vi "test2.vi"() -> ()   [LabVIEW 2013]
uses:
  <vilib>/Utility/file.llb/Write To Spreadsheet File (string).vi
panel:
  out "appended path":path
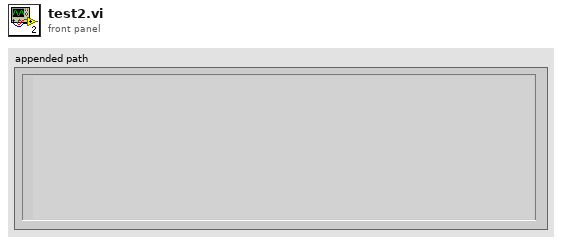
[diagram p1: front panel]
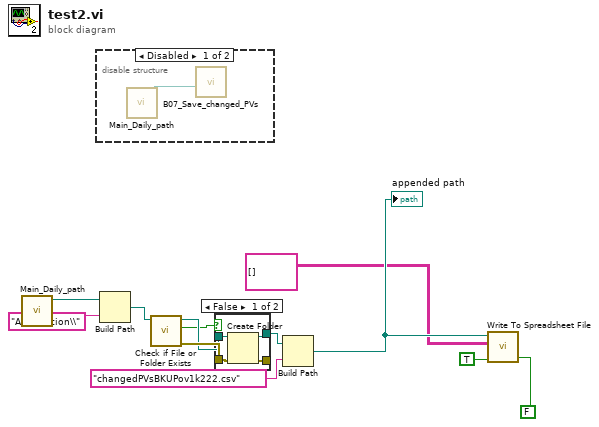
[diagram p0: block diagram]
diagram:
  n1 = call "Main_Daily_path.vi"() -> ("Directory path"=w6:path)  [unwired: 10 in, 1 out]
  n2 = disable-structure shown="Disabled" {
    frame Disabled {
      n3 = call "Main_Daily_path.vi"() -> ("Directory path"=w13:path)  [unwired: 10 in, 1 out]
      n4 = call "B07_Save_changed_PVs.vi"("Directory Path"=w13) -> ()  [unwired: 9 in, 2 out]
    }
    frame Enabled {
    }
  }
  n5 = Build Path(base path=w6, name or relative path="Association\\" ("string")) -> (appended path=w10:path)
  n6 = call <vilib>:"Check if File or Folder Exists.vi"("path"=w10) -> ("error out"=w9:errorcluster, "file or folder exists?"=w7:bool, "dup path"=w8:path)  [unwired: 8 in]
  n7 = case shown="False" w7 {
    tunnel: w8 -> [w17 w18]
    tunnel: [w16 w19] -> _
    tunnel: w9 -> [w15 w19]
    tunnel: [w14 w18] -> w11
    frame False {
      n8 = Create Folder(path (use dialog)=w17, error in=w15) -> (created path=w14:path, error out=w16:errorcluster)  [unwired: 1 in, 1 out]
    }
    frame True {
    }
  }
  n9 = Build Path(base path=w11, name or relative path="changedPVsBKUPov1k222.csv" ("string")) -> (appended path=w2:path)
  "appended path" <- w2
  n10 = call-poly <vilib>:"Write To Spreadsheet File.vi"("transpose? (no:F)"=FALSE, "append to file? (new file:F)"=TRUE, "2D data"=string[][] [], "file path (dialog if empty)"=w2) -> ()  [unwired: 4 in, 1 out]
